vi "Integer Wavelet Transform on 1D Signal.vi"() -> ()   [LabVIEW 2023]
doc: "This example shows how to perform the integer wavelet transform (IWT) on an integer signal with the WA Integer Wavelet Transform VI.\n\n<b>Instructions:</b>\n1) Run this VI.\n2) Specify a <b>Signal Type</b>.\n3) Change the <b>Wavelet</b>, <b>Levels</b>, and <b>Extension</b> settings and observe the <b>IWT Coefficients</b>.\n4) Browse the Block Diagram of this example to learn how to analyze an integer signal by using the integer wavelet transform and how to reconstruct the integer signal by using the inverse integer wavelet transform."
uses:
  <vilib>/addons/Wavelet Analysis/discrete wavelet transform.llb/WA 1D Integer Wavelet Transform.vi
  <vilib>/addons/Wavelet Analysis/discrete wavelet transform.llb/WA Inverse 1D Integer Wavelet Transform.vi
  <vilib>/Analysis/NI_AALPro.lvlib
  <vilib>/addons/_Advanced Signal Processing/NI_AdvSigProcWA.lvlib
panel:
  in  "Signal Type":T1(ring)
  in  "stop":bool
  in  "Wavelet":u16(ring)=13 items=["Haar"=13, "bior2_2"=16, "bior4_4 (FBI)"=25]
  out "IWT Coefficients":i32[](graph)
  out "Reconstruct Signal":i32[](graph)
  out "Signal":i32[](graph)
  in  "Extension":u16(ring)=1 items=["Zero padding", "Symmetric", "Periodic"]
  in  "Levels":i32=9
  # "Overview: Shows how to perform the integer wavelet transform (IWT) on an integer signal with the WA Integer Wavelet Transform VI.\nRequirements: LabVIEW Full Development System, Advanced Signal Processing Toolkit\nInstructions: \n1. Run this VI.  Specify a Signal Type.\n2. Change the Wavelet, Levels, and Extension settings and observe the IWT Coefficients.\n3. Browse the block diagram of this example to learn how to analyze an integer signal by using the integer wavelet transform and how to reconstruct the integer signal by using the inverse integer wavelet transform.\n4. Click Stop to stop the VI."
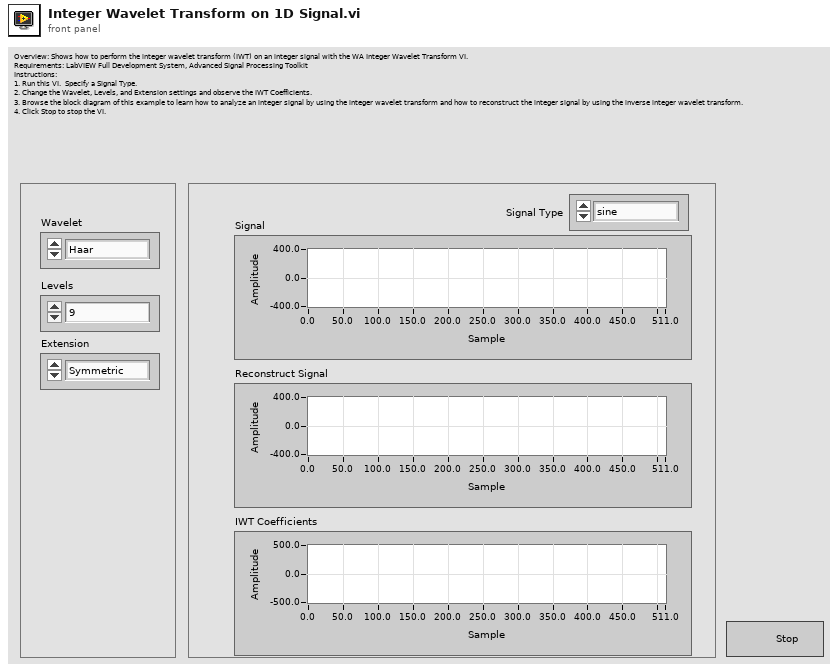
[diagram p1: front panel]
types:
  T1 = enum16{"sine", "cosine", "triangle", "square", "sawtooth", "increasing ramp", "decreasing ramp"}
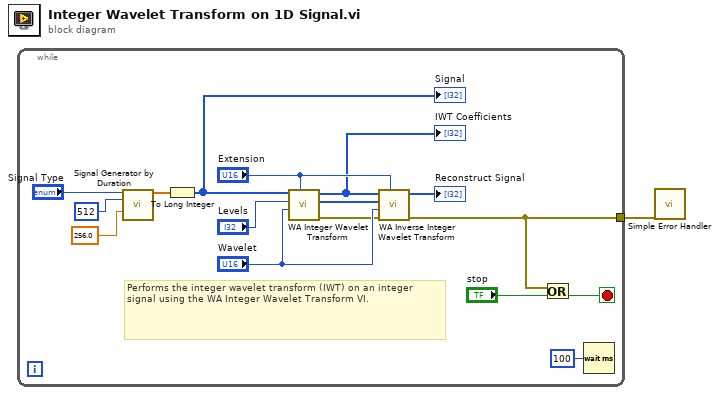
[diagram p0: block diagram]
diagram:
  n1 = while {
    tunnel: [w3] -> w1
    stop <- w5 stop-if-true
    # "Performs the integer wavelet transform (IWT) on an integer signal using the WA Integer Wavelet Transform VI."
    n2 = call <vilib>:"Signal Generator by Duration.vi"("signal type"="Signal Type", "# of samples"=512, "amplitude"=256.0) -> ("signal"=w15:dbl[])  [unwired: 4 in, 8 out]
    n3 = To Long Integer(number=w15) -> (32bit integer=w11:i32[])
    "Signal" <- w11
    n4 = call-poly <vilib>:"WA Integer Wavelet Transform.vi"("extension"="Extension", "wavelet"="Wavelet", "levels"="Levels", "signal"=w11) -> ("error out"=w7:errorcluster, "length"=w13:i32[], "IWT coef"=w9:i32[])  [unwired: 1 in, 4 out]
    "IWT Coefficients" <- w9
    n5 = call-poly <vilib>:"WA Inverse Integer Wavelet Transform.vi"("extension"="Extension", "error in (no error)"=w7, "wavelet"="Wavelet", "length"=w13, "IWT coef"=w9) -> ("error out"=w3:errorcluster, "signal"=→"Reconstruct Signal":i32[])  [unwired: 5 out]
    n6 = Or(x=w3, y="stop") -> (x .or. y?=w5:bool)
    n7 = Wait (ms)(milliseconds to wait=u32 100) -> ()  [unwired: 1 out]
  }
  n8 = call <vilib>:"Simple Error Handler.vi"("error in (no error)"=w1) -> ()  [unwired: 1 in, 8 out]
